vi "Write to File.vi"(8 "error in":errorcluster, 10 "File Actor In":refnum<class "File Actor.lvclass">, 11 "Exe Write in":refnum<class "Exe Write.lvclass">) -> (0 "error out":errorcluster, 2 "File Actor Out":refnum<class "File Actor.lvclass">)   [LabVIEW 2017, in "File Library.lvlib" / "Exe Write.lvclass"]
doc: "This is the sould of the execution method and the only VI that should be overriden. This is where we expect the file to be written."
uses:
  Exe Write.lvclass
  File Actor.lvclass
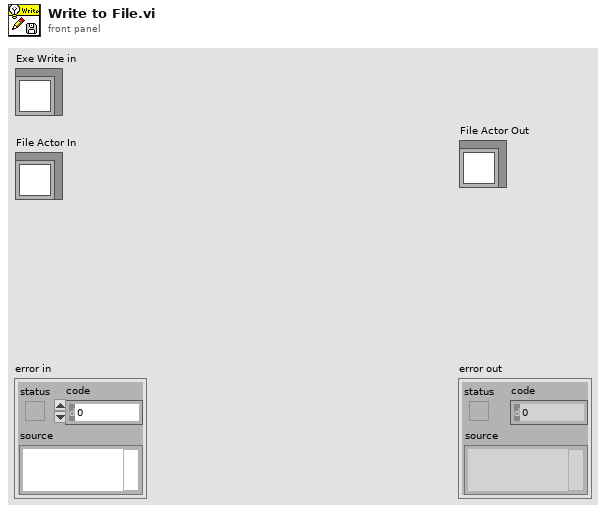
[diagram p1: front panel]
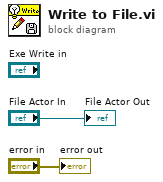
[diagram p0: block diagram]
diagram:
  "error out" <- "error in"
  "File Actor Out" <- "File Actor In"
